vi "lab1_Shimeng_LI.vi"() -> ()   [LabVIEW 2014]
uses:
  <vilib>/Instr/_visa.llb/VISA Configure Serial Port (Instr).vi
  <vilib>/Utility/file.llb/Read From Spreadsheet File (DBL).vi
  <vilib>/imath/engines/lvmath2/RunTimeEngine/NodeEndStatement/NIMS_NodeEndStatement_Output.vi
  <instcachedir>/0/NIMS_NodeEndStatement_Output_53EC0D466D134D7ABD903AC30B43404B.lvgen/NIMS_NodeEndStatement_Output_53EC0D466D134D7ABD903AC30B43404B_001.vi
  <vilib>/imath/engines/lvmath2/RunTimeEngine/ErrorHandling/NIMS_Finalize Error.vi
  <vilib>/Utility/file.llb/Write To Spreadsheet File (DBL).vi
panel:
  out "List with new object points":dbl[][](array[numeric])
  in  "file path for calculated object points":path
  out "Response 2":string
  in  "Request 2":string
  in  "Array":dbl[][](array[numeric])
  out "New Object Points Global":dbl[](array[numeric])
  in  "Stop Everything 2":bool
  in  "Send Request 2":bool
  in  "Timeout [ms] 2":u32=5000
  out "resY":dbl[](array[numeric])
  out "resX":dbl[](array[numeric])
  out "Current Coordinate":dbl[](array[numeric])
  out "Global Coordinates":dbl[][](array[numeric]) format="%0.3f"
  in  "file path (dialog if empty)":path
  in  "calculate transformation":bool
  out "Local Coordinate":dbl[][](array[numeric])
  in  "delete":bool
  in  "delete row":i32
  out "Local  Coordinates Measurement":dbl[][](array[numeric])
  in  "Timeout [ms]":u32=5000
  in  "Stop Everything":bool
  in  "Send Request":bool
  out "Answer":string
  in  "Request":string
  in  "parity (0:none)":enum16{"None", "Odd", "Even", "Mark", "Space"}(ring)
  in  "data bits (8)":u16=8 min=5 max=8 step=1
  in  "baud rate (9600)":u32=9600
  in  "VISA resource name":refnum<visa-resource-name>
  # "Communication Parameter"
  # "Measurement of the local coordinates"
  # "First Step: measure local\ncoordinates of known \npoints"
  # "Helmert  Transformation"
  # "Second Step: calculate a\nHelmert Transformation"
  # "Third Step: measure new \nobject points in global \nreference system"
  # "Measure and save new object points with global  coordinates"
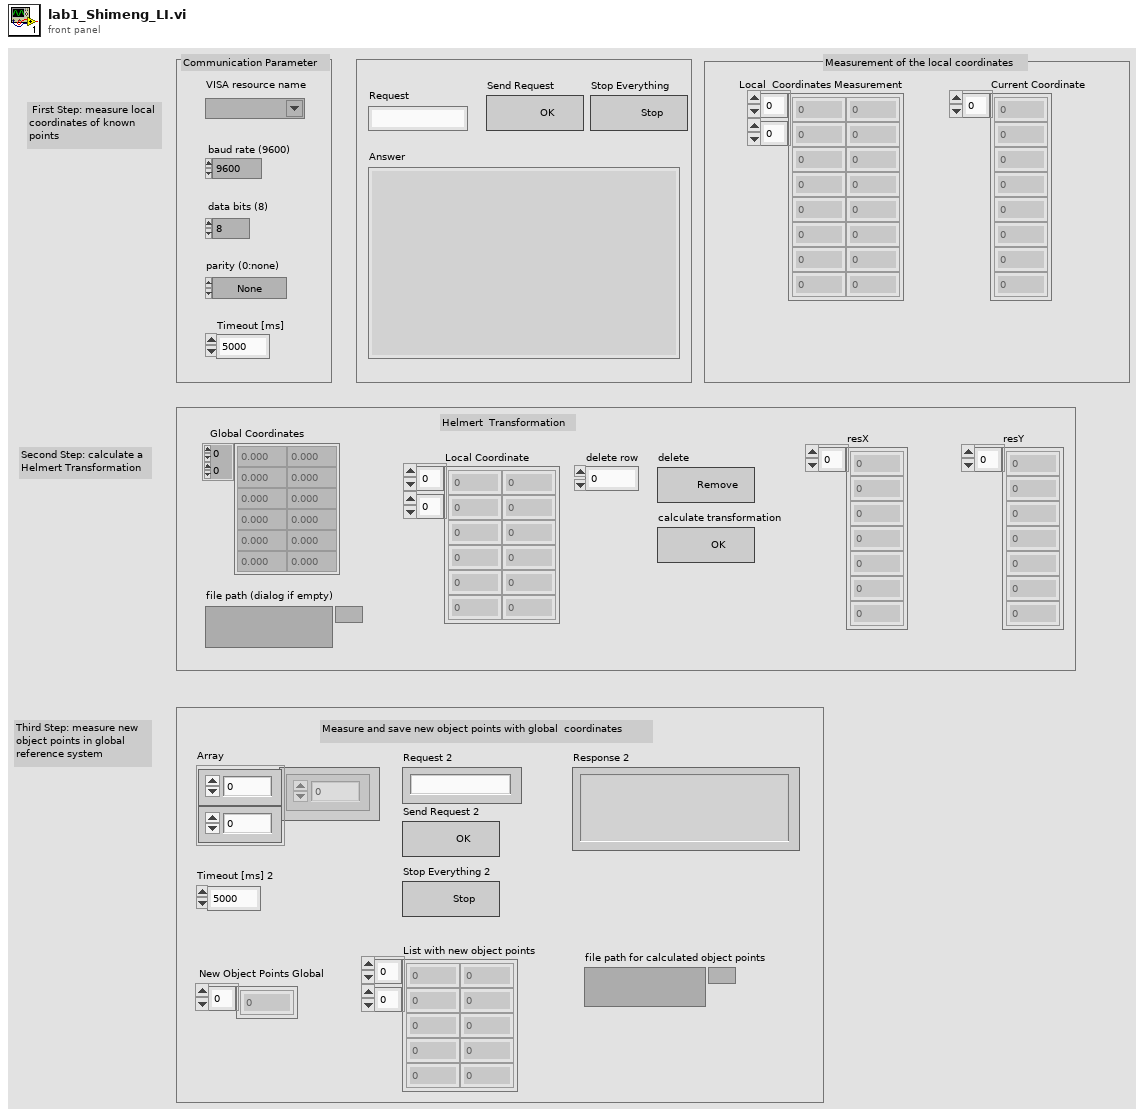
[diagram p1: front panel]
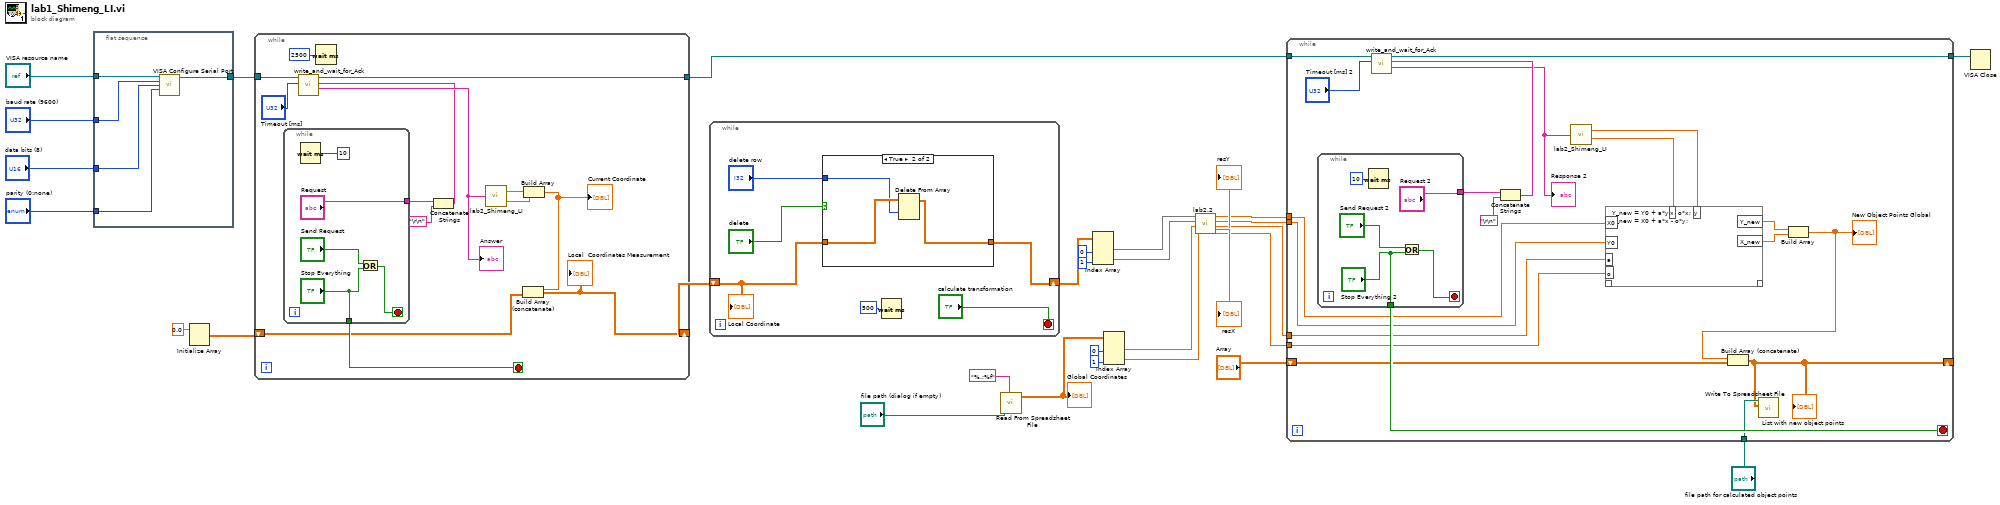
[diagram p0: block diagram]
diagram:
  n1 = flat-sequence {
    tunnel: "VISA resource name" -> [w35]
    tunnel: "baud rate (9600)" -> [w34]
    tunnel: "data bits (8)" -> [w33]
    tunnel: "parity (0:none)" -> [w32]
    tunnel: [w31] -> w26
    frame #0 {
      n2 = call-poly "VISA Configure Serial Port"("VISA resource name"=w35, "baud rate (9600)"=w34, "data bits (8)"=w33, "parity (0:none)"=w32) -> ("VISA resource name out"=w31:refnum<visa-resource-name>)  [unwired: 10 in, 1 out]
    }
  }
  n3 = Initialize Array(0.0 ("element")) -> (w1:dbl[][])  [unwired: 2 in]
  n4 = while {
    tunnel: [w49] -> w10
    tunnel: w26 -> [w48]
    shift-right: [w42] -> w25
    shift-left: w1 -> [w43]
    stop <- w47 stop-if-true
    n5 = while {
      tunnel: ["Stop Everything"] -> w47
      tunnel: ["Request"] -> w37
      stop <- w52 stop-if-true
      n6 = Wait (ms)(milliseconds to wait=u32 10) -> ()  [unwired: 1 out]
      n7 = Or(x="Send Request", y="Stop Everything") -> (x .or. y?=w52:bool)
    }
    n8 = Wait (ms)(milliseconds to wait=u32 2500) -> ()  [unwired: 1 out]
    n9 = Concatenate Strings(w37, "\r\n") -> (w38:string)
    n10 = call "write_and_wait_for_Ack.vi"("request"=w38, "Timeout [ms]"="Timeout [ms]", "VISA resource name"=w48) -> ("result"=w45:string, "VISA resource name out"=w49:refnum<visa-resource-name>)  [unwired: 4 in, 1 out]
    "Answer" <- w45
    n11 = call "lab2_Shimeng_LI.vi"("String Input"=w45) -> ("x local"=w44:dbl, "y local"=w41:dbl)
    n12 = Build Array(w44, w41) -> (w40:dbl[])
    "Current Coordinate" <- w40
    n13 = Build Array (concatenate)(w40, w43) -> (w42:dbl[][])
    "Local  Coordinates Measurement" <- w42
  }
  n14 = while {
    shift-right: [w58] -> w17
    shift-left: w25 -> [w59]
    stop <- "calculate transformation" stop-if-true
    n15 = case shown="True" "delete" {
      tunnel: w59 -> [w61 w64]
      tunnel: [w61 w62] -> w58
      tunnel: "delete row" -> [_ w63]
      frame False {
      }
      frame True {
        n16 = Delete From Array(array=w64, index (row)=w63) -> (array with subset deleted=w62:dbl[][])  [unwired: 2 in, 1 out]
      }
    }
    n17 = Wait (ms)(milliseconds to wait=u32 500) -> ()  [unwired: 1 out]
    "Local Coordinate" <- w59
  }
  n18 = call-poly <vilib>:"Read From Spreadsheet File.vi"("format (%.3f)"="%.;%f", "file path (dialog if empty)"="file path (dialog if empty)") -> ("all rows"=w22:dbl[][])  [unwired: 5 in, 4 out]
  "Global Coordinates" <- w22
  n19 = Index Array(array=w17, index (col) #1=0 ("disabled index (col)"), index (col) #2=1 ("index (col)")) -> (element #1=w14:dbl[], element #2=w13:dbl[])  [unwired: 2 in]
  n20 = Index Array(array=w22, index (col) #1=0 ("disabled index (col)"), index (col) #2=1 ("disabled index (col)")) -> (element #1=w19:dbl[], element #2=w18:dbl[])  [unwired: 2 in]
  n21 = call "lab2.2.vi"("y global"=w18, "x global"=w19, "y local"=w13, "x local"=w14) -> ("o"=w5:dbl, "a"=w6:dbl, "Y0"=w7:dbl, "X0"=w8:dbl, "resY"=→"resY":dbl[], "resX"=→"resX":dbl[])  [unwired: 2 in]
  n22 = while {
    tunnel: w10 -> [w84]
    tunnel: [w83] -> w9
    tunnel: w8 -> [w77]
    tunnel: w7 -> [w76]
    tunnel: w6 -> [w75]
    tunnel: w5 -> [w74]
    shift-right: [w66] -> _
    shift-left: "Array" -> [w65]
    tunnel: "file path for calculated object points" -> [w67]
    stop <- w80 stop-if-true
    n23 = while {
      tunnel: ["Stop Everything 2"] -> w80
      tunnel: ["Request 2"] -> w70
      stop <- w135 stop-if-true
      n24 = Wait (ms)(milliseconds to wait=u32 10) -> ()  [unwired: 1 out]
      n25 = Or(x="Send Request 2", y="Stop Everything 2") -> (x .or. y?=w135:bool)
    }
    n26 = Concatenate Strings(w70, "\r\n") -> (w69:string)
    n27 = call "write_and_wait_for_Ack.vi"("request"=w69, "Timeout [ms]"="Timeout [ms] 2", "VISA resource name"=w84) -> ("result"=w68:string, "VISA resource name out"=w83:refnum<visa-resource-name>)  [unwired: 4 in, 1 out]
    "Response 2" <- w68
    n28 = call "lab2_Shimeng_LI.vi"("String Input"=w68) -> ("x local"=w78:dbl, "y local"=w79:dbl)
    n29 = mathscript code="Y_new = Y0 + a*y + o*x;\nX_new = X0 + a*x - o*y;"("X0"=w77, "Y0"=w76, "a"=w75, "o"=w74, "x"=w78, "y"=w79) -> ("Y_new"=w73:dbl, "X_new"=w72:dbl)  [unwired: 1 in, 1 out]
    n30 = Build Array(w73, w72) -> (w71:dbl[])
    "New Object Points Global" <- w71
    n31 = Build Array (concatenate)(w71, w65) -> (w66:dbl[][])
    "List with new object points" <- w66
    n32 = call-poly <vilib>:"Write To Spreadsheet File.vi"("2D data"=w66, "file path (dialog if empty)"=w67) -> ()  [unwired: 6 in, 1 out]
  }
  n33 = VISA Close(VISA resource name=w9) -> ()  [unwired: 1 in, 1 out]
